vi "Controller Revised.vi"() -> ()   [LabVIEW 2018]
uses:
  <vilib>/DAQmx/read.llb/DAQmx Read (Analog DBL 1Chan 1Samp).vi
  <vilib>/DAQmx/write.llb/DAQmx Write (Digital Bool 1Line 1Point).vi
  <vilib>/DAQmx/create/channels.llb/DAQmx Create Channel (DO-Digital Output).vi
  <vilib>/DAQmx/miscellaneous.llb/DAQmx Fill In Error Info.vi
  <vilib>/DAQmx/create/channels.llb/DAQmx Create Channel (AI-Temperature-Thermocouple).vi
  <vilib>/addons/control/pid/pid.llb/PID Gain Schedule (DBL).vi
  <vilib>/addons/control/pid/pid.llb/PID Advanced (DBL).vi
  <vilib>/addons/control/pid/NI_PID_pid.lvlib
panel:
  out "SP:":dbl(slide)=60.7843137254902 min=0.0 max=0.0 scale=0.0..100.0
  out "PV:":dbl(slide) scale=0.0..100.0
  out "MV:":dbl(slide)=18.78965245852964 scale=-100.0..100.0
  in  "Sampling Time dt (s)":dbl=0.05 min=0.001 step=0.01 format="%#.3p"
  out "PV Setpoint Output":cluster{"initial PV":dbl, "setpoint":dbl}(graph)={"initial PV"=22.75459115919792, "setpoint"=26.050000000000235}
  in  "Stop":bool
  in  "setpoint profile":cluster{"time (s)":dbl, "setpoint":dbl}[](array[cluster])
  out "Profile Elapsed Time (s)":dbl=15.000000000000078 format="%.3f"
  in  "Reinitialize Profile":bool
  in  "PID gain schedule":T1(array[cluster])=[{"PID gains"={"proportional gain (Kc)"=1.0, "integral time (Ti, min)"=0.01, "derivative time (Td, min)"=0.0}, "max value"=100.0}] {"max value" format="%.2f"; "PID gains"."derivative time (Td, min)" format="%.6f"; "PID gains"."integral time (Ti, min)" format="%.6f"; "PID gains"."proportional gain (Kc)" format="%.6f"}
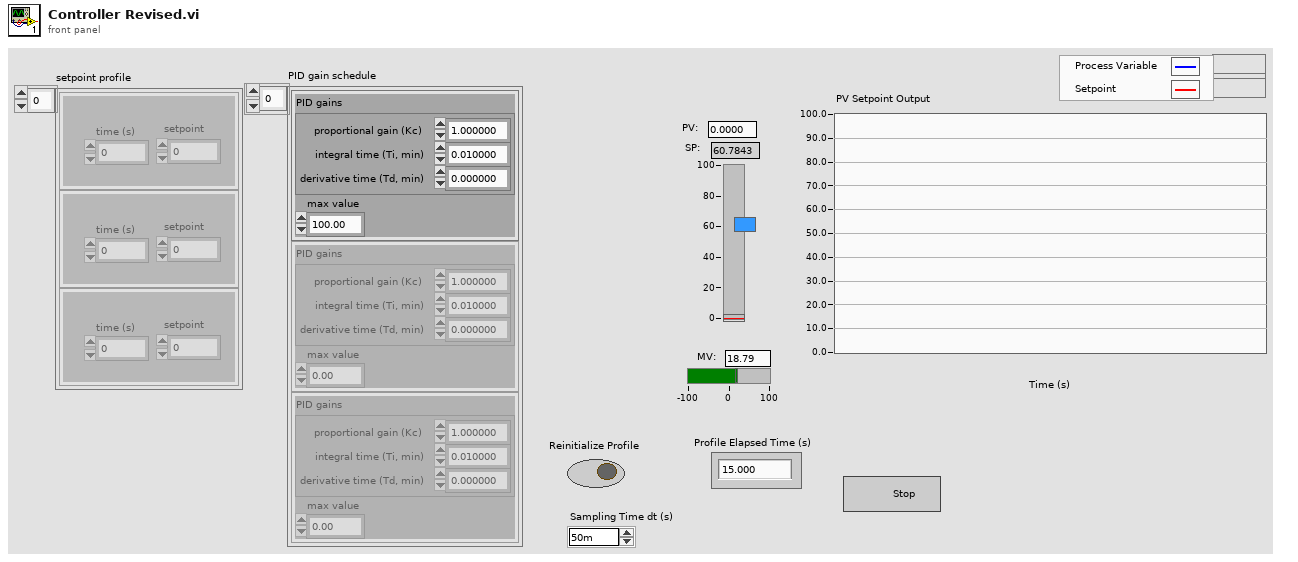
[diagram p1: front panel]
types:
  T1 = cluster{"PID gains":cluster{"proportional gain (Kc)":dbl, "integral time (Ti, min)":dbl, "derivative time (Td, min)":dbl}, "max value":dbl}[]
  T2 = cluster{"proportional gain (Kc)":dbl, "integral time (Ti, min)":dbl, "derivative time (Td, min)":dbl}
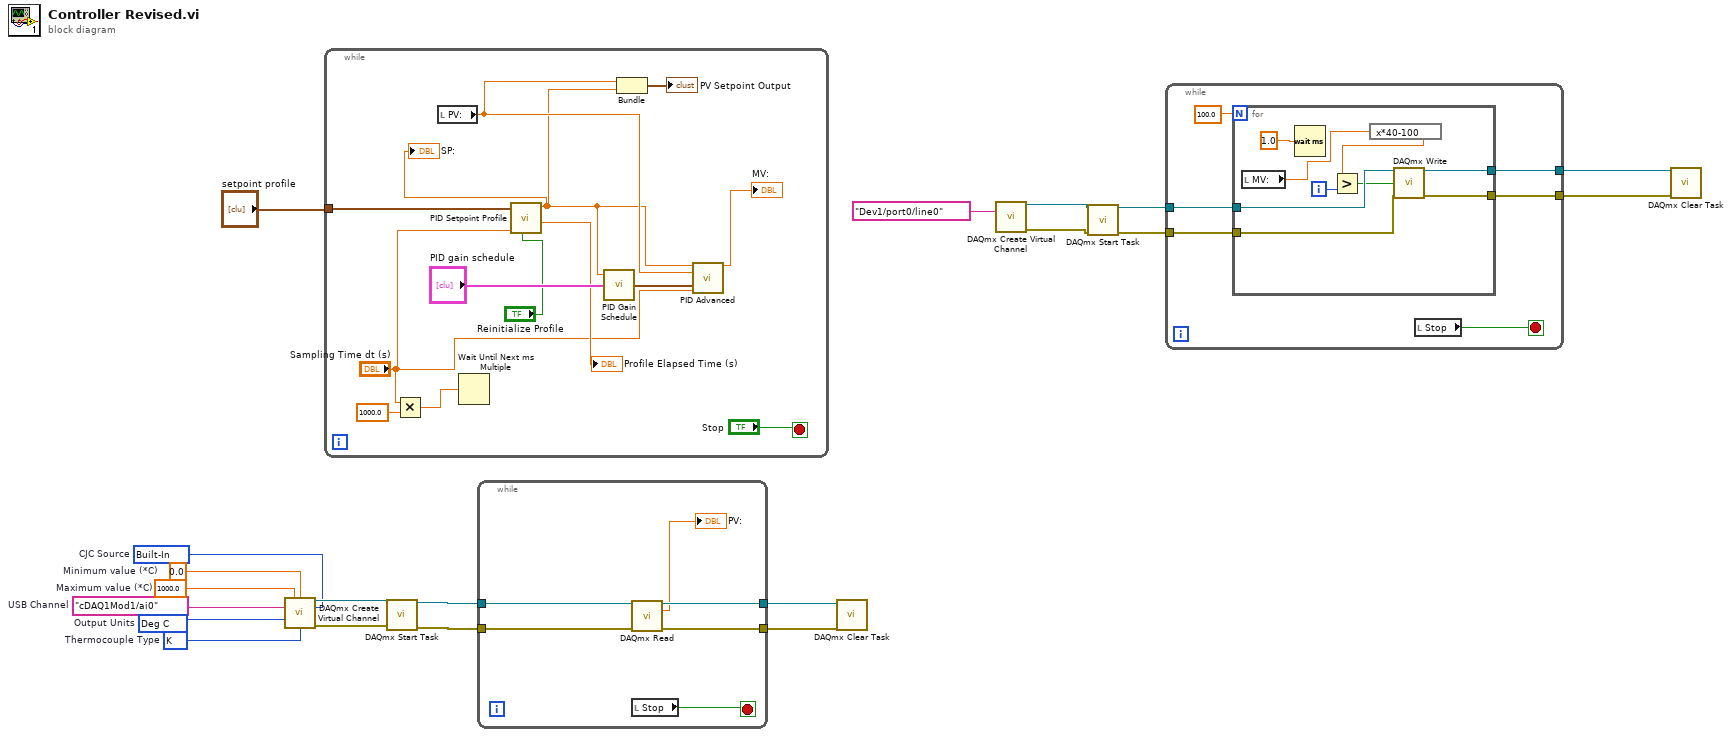
[diagram p0: block diagram]
diagram:
  w5 = 10143 items=["Deg C"=10143, "Deg F"=10144, "Kelvins"=10325, "Deg R"=10145, "From Custom Scale"=10065]  # Output Units
  w9 = 10073 items=["J"=10072, "K"=10073, "N"=10077, "R"=10082, "S"=10085, "T"=10086, "B"=10047, "E"=10055]  # Thermocouple Type
  w6 = tag "cDAQ1Mod1/ai0"  # USB Channel
  w7 = 1000.0  # Maximum value (*C)
  w8 = 0.0  # Minimum value (*C)
  w4 = 10200 items=["Built-In"=10200, "Constant Value"=10116, "Channel"=10113]  # CJC Source
  n1 = call-poly <vilib>:"DAQmx Create Virtual Channel.vi"("maximum value"=w7, "minimum value"=w8, "physical channels"=w6, "cjc source"=w4, "units"=w5, "thermocouple type"=w9) -> ("task out"=w13:refnum<k21>, "error out"=w11:errorcluster)  [unwired: 8 in]
  n2 = while {
    tunnel: "setpoint profile" -> [w31]
    stop <- "Stop" stop-if-true
    n3 = Multiply(x="Sampling Time dt (s)", y=1000.0) -> (x*y=w26:dbl)
    n4 = local read "PV:"() -> (w22:dbl)
    n5 = Wait Until Next ms Multiple(millisecond multiple=w26) -> ()  [unwired: 1 out]
    n6 = call <vilib>:"PID Setpoint Profile.vi"("reinitialize? (F)"="Reinitialize Profile", "dt (s)"="Sampling Time dt (s)", "setpoint profile"=w31) -> ("elapsed time (s)"=→"Profile Elapsed Time (s)":dbl, "setpoint"=w21:dbl)  [unwired: 3 in, 2 out]
    "SP:" <- w21
    n7 = call-poly <vilib>:"PID Gain Schedule.vi"("PID gain schedule"="PID gain schedule", "gain scheduling value"=w21) -> ("PID gains out"=w33:T2)  [unwired: 2 in, 1 out]
    n8 = Bundle("PV:"=w22, "setpoint"=w21) -> (→"PV Setpoint Output":cluster{"PV:":dbl, "setpoint":dbl})  [unwired: 1 in]
    n9 = call-poly <vilib>:"PID Advanced.vi"("setpoint"=w21, "process variable"=w22, "PID gains"=w33, "dt (s)"="Sampling Time dt (s)") -> ("output"=→"MV:":dbl)  [unwired: 10 in, 1 out]
  }
  n10 = call <vilib>:"DAQmx Start Task.vi"("task/channels in"=w13, "error in"=w11) -> ("task out"=w12:refnum<k21>, "error out"=w10:errorcluster)  [unwired: 12 in]
  n11 = while {
    tunnel: w12 -> [w39]
    tunnel: w10 -> [w38]
    tunnel: [w37] -> w3
    tunnel: [w36] -> w2
    stop <- w34 stop-if-true
    n12 = call-poly <vilib>:"DAQmx Read.vi"("task/channels in"=w39, "error in"=w38) -> ("task out"=w37:refnum<k21>, "data"=→"PV:":dbl, "error out"=w36:errorcluster)  [unwired: 11 in]
    n13 = local read "Stop"() -> (w34:bool)
  }
  n14 = call <vilib>:"DAQmx Clear Task.vi"("task in"=w3, "error in"=w2) -> ()  [unwired: 13 in, 1 out]
  n15 = call-poly <vilib>:"DAQmx Create Virtual Channel.vi"("lines"=tag "Dev1/port0/line0") -> ("task out"=w18:refnum<k21>, "error out"=w17:errorcluster)  [unwired: 13 in]
  n16 = call <vilib>:"DAQmx Start Task.vi"("task/channels in"=w18, "error in"=w17) -> ("task out"=w16:refnum<k21>, "error out"=w15:errorcluster)  [unwired: 12 in]
  n17 = while {
    tunnel: [w44] -> w20
    tunnel: [w43] -> w19
    tunnel: w16 -> [w42]
    tunnel: w15 -> [w41]
    stop <- w40 stop-if-true
    n18 = for {
      N: 100.0 -> [_]
      tunnel: [w48] -> w44
      tunnel: [w52] -> w43
      tunnel: w42 -> [w51]
      tunnel: w41 -> [w50]
      i -> [w54]
      n19 = local read "MV:"() -> (w46:dbl)
      n20 = Wait (ms)(milliseconds to wait=1.0) -> ()  [unwired: 1 out]
      n21 = expression code="x*40-100"(w46) -> (w49:dbl)
      n22 = Greater?(x=w49, y=w54) -> (0:w47:bool)
      n23 = call-poly <vilib>:"DAQmx Write.vi"("task/channels in"=w51, "data"=w47, "error in"=w50) -> ("task out"=w48:refnum<k21>, "error out"=w52:errorcluster)  [unwired: 10 in, 1 out]
    }
    n24 = local read "Stop"() -> (w40:bool)
  }
  n25 = call <vilib>:"DAQmx Clear Task.vi"("task in"=w20, "error in"=w19) -> ()  [unwired: 13 in, 1 out]
